vi "Update_TS_WIP.vi"(8 "error in (no error)":errorcluster, 10 "WIP Limit":T2, 11 "Refnum in":T1) -> (0 "error out":errorcluster, 3 "Refnum out":T1)   [LabVIEW 2020]
uses:
  <vilib>/addons/database/Connection.llb/Conn ObjectReference.ctl
  Controls/WIP Limit.ctl
  Controls/WIP_old.ctl
  <vilib>/addons/database/Connection.llb/Conn Execute.vi
  <vilib>/addons/database/Recordset.llb/Rec Destroy - Connection.vi
  <vilib>/addons/database/NI_Database_API.lvlib
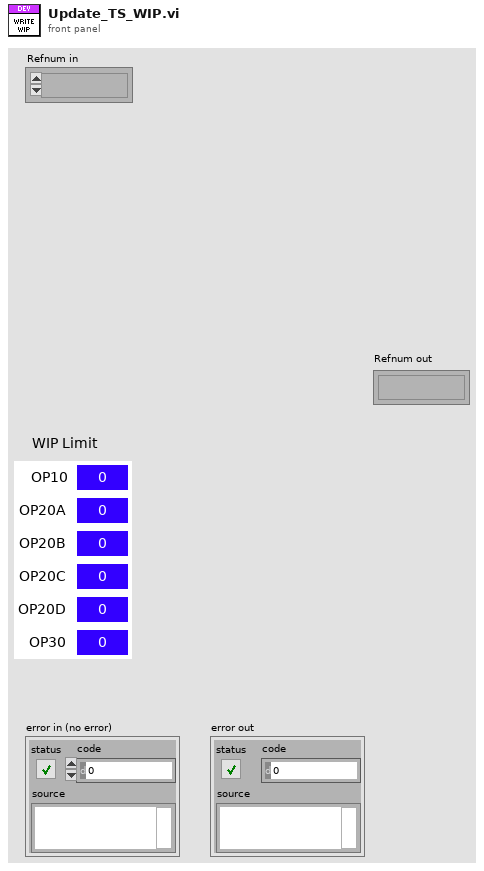
[diagram p1: front panel]
types:
  T1 = typedef "NI_Database_API.lvlib/Conn ObjectReference.ctl" = refnum<k1>
  T2 = typedef "WIP Limit.ctl" = cluster{"OP10":T3, "OP20A":T3, "OP20B":T3, "OP20C":T3, "OP20D":T3, "OP30":T3}
  T3 = typedef "WIP_old.ctl" = i64
  T4 = typedef "NI_Database_API.lvlib/Rec ObjectReference.ctl" = refnum<k1>
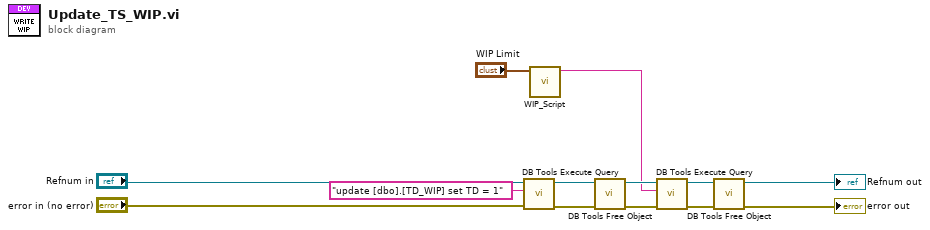
[diagram p0: block diagram]
diagram:
  n1 = call-poly <vilib>:"DB Tools Execute Query.vi"("error in (no error)"="error in (no error)", "SQL query"="update [dbo].[TD_WIP] set TD = 1", "connection reference"="Refnum in") -> ("error out"=w11:errorcluster, "recordset reference"=w10:T4)  [unwired: 5 in]
  n2 = call "WIP_Script.vi"("WIP Limit"="WIP Limit") -> ("iNSERT Script"=w6:string)  [unwired: 10 in]
  n3 = call-poly <vilib>:"DB Tools Free Object.vi"("error in (no error)"=w11, "recordset reference"=w10) -> ("error out"=w13:errorcluster, "connection reference"=w12:T1)  [unwired: 8 in]
  n4 = call-poly <vilib>:"DB Tools Execute Query.vi"("error in (no error)"=w13, "SQL query"=w6, "connection reference"=w12) -> ("error out"=w3:errorcluster, "recordset reference"=w4:T4)  [unwired: 5 in]
  n5 = call-poly <vilib>:"DB Tools Free Object.vi"("error in (no error)"=w3, "recordset reference"=w4) -> ("error out"=→"error out":errorcluster, "connection reference"=→"Refnum out":T1)  [unwired: 8 in]
